vi "배열 글로벌.vi"() -> ()   [LabVIEW 2014]
panel:
  in  "배열":dbl[](array[numeric])
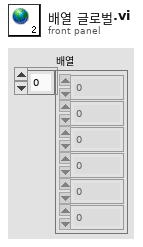
[diagram p1: front panel]
diagram:
